vi "Drive type properties.vi"(1 "Type":T1) -> (3 "Nominal resolution":i32, 4 "Effective resolution":dbl, 5 "Rotary":bool, 6 "Speed multiplier":dbl)   [LabVIEW 2019]
uses:
  Axis enum.ctl
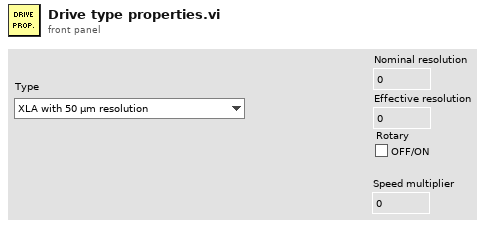
[diagram p1: front panel]
types:
  T1 = typedef "Axis enum.ctl" = enum16{"XLA with 50 µm resolution", "XLA with 10 µm resolution", "XLA with 1250 nm resolution", "XLA with 312 nm resolution", "XLA with 78 nm resolution", "XLS with 1250 nm resolution", "XLS with 312 nm resolution", "XLS with 78nm resolution", "XLS with 5nm resolution", "XLS with 1 nm resolution", "XRT-A with 109 µrad resolution", "XRT-U-30 with 109 µrad resolution", "XRT-U-30 with 49 µrad resolution", "XRT-U-30 with 19 µrad resolution", "XRT-U-30 with 3 µrad resolution", "XRT-U-40 with 109 µrad resolution", "XRT-U 40 with 49 µrad resolution", "XRT-U-40 with 19 µrad resolution", "XRT-U-40 with 3 µrad resolution", "XRT-U-60 with 109 µrad resolution", "XRT-U-60 with 49 µrad resolution", "XRT-U-60 with 19 µrad resolution", "XRT-U-60 with 3 µrad resolution"}
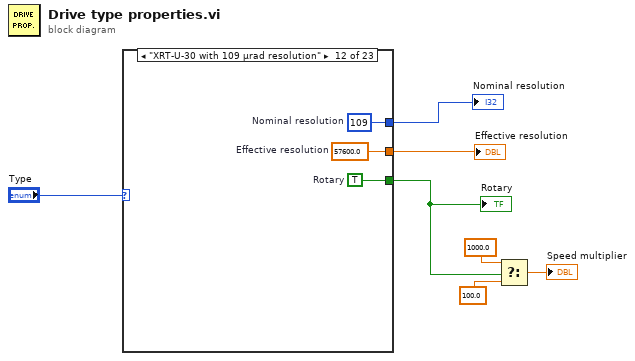
[diagram p0: block diagram]
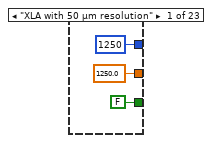
[diagram p2: hidden frame]
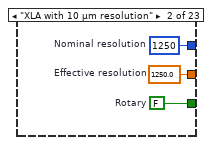
[diagram p3: hidden frame]
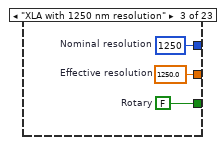
[diagram p4: hidden frame]
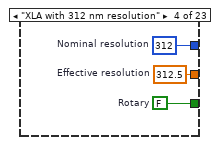
[diagram p5: hidden frame]
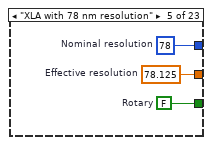
[diagram p6: hidden frame]
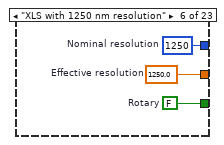
[diagram p7: hidden frame]
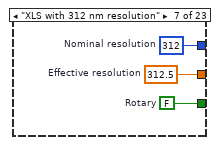
[diagram p8: hidden frame]
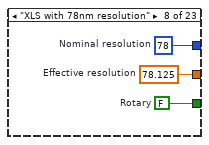
[diagram p9: hidden frame]
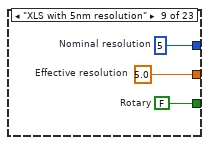
[diagram p10: hidden frame]
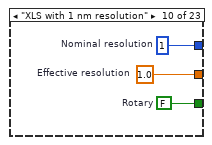
[diagram p11: hidden frame]
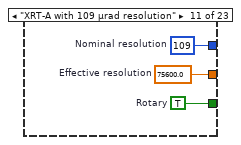
[diagram p12: hidden frame]
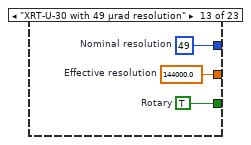
[diagram p13: hidden frame]
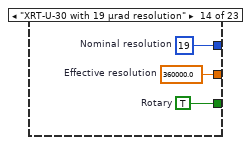
[diagram p14: hidden frame]
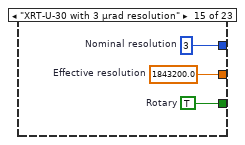
[diagram p15: hidden frame]
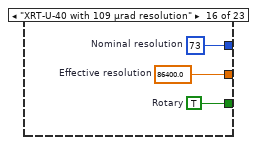
[diagram p16: hidden frame]
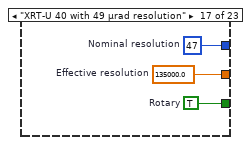
[diagram p17: hidden frame]
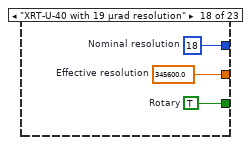
[diagram p18: hidden frame]
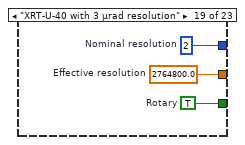
[diagram p19: hidden frame]
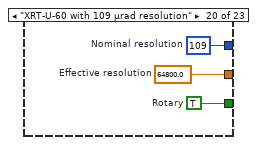
[diagram p20: hidden frame]
diagram:
  n1 = case shown="\"XRT-U-30 with 109 µrad resolution\"" "Type" {
    tunnel: [1250 ("Nominal resolution") w13 w16 w19 w22 w25 w28 w31 w34 w37 w40 w43 w46 w49 w52 w55 w58 w61 w64 w67 w70 w73 w76] -> w6
    tunnel: [1250.0 ("Effective resolution") w12 w15 w18 w21 w24 w27 w30 w33 w36 w39 w42 w45 w48 w51 w54 w57 w60 w63 w66 w69 w72 w75] -> w5
    tunnel: [FALSE ("Rotary") w11 w14 w17 w20 w23 w26 w29 w32 w35 w38 w41 w44 w47 w50 w53 w56 w59 w62 w65 w68 w71 w74] -> w4
    frame "XLA with 50 µm resolution" {
    }
    frame "XLA with 10 µm resolution" {
      w11 = FALSE  # Rotary
      w12 = 1250.0  # Effective resolution
      w13 = 1250  # Nominal resolution
    }
    frame "XLA with 1250 nm resolution" {
      w14 = FALSE  # Rotary
      w15 = 1250.0  # Effective resolution
      w16 = 1250  # Nominal resolution
    }
    frame "XLA with 312 nm resolution" {
      w17 = FALSE  # Rotary
      w18 = 312.5  # Effective resolution
      w19 = 312  # Nominal resolution
    }
    frame "XLA with 78 nm resolution" {
      w20 = FALSE  # Rotary
      w21 = 78.125  # Effective resolution
      w22 = 78  # Nominal resolution
    }
    frame "XLS with 1250 nm resolution" {
      w23 = FALSE  # Rotary
      w24 = 1250.0  # Effective resolution
      w25 = 1250  # Nominal resolution
    }
    frame "XLS with 312 nm resolution" {
      w26 = FALSE  # Rotary
      w27 = 312.5  # Effective resolution
      w28 = 312  # Nominal resolution
    }
    frame "XLS with 78nm resolution" {
      w29 = FALSE  # Rotary
      w30 = 78.125  # Effective resolution
      w31 = 78  # Nominal resolution
    }
    frame "XLS with 5nm resolution" {
      w32 = FALSE  # Rotary
      w33 = 5.0  # Effective resolution
      w34 = 5  # Nominal resolution
    }
    frame "XLS with 1 nm resolution" {
      w35 = FALSE  # Rotary
      w36 = 1.0  # Effective resolution
      w37 = 1  # Nominal resolution
    }
    frame "XRT-A with 109 µrad resolution" {
      w38 = TRUE  # Rotary
      w39 = 75600.0  # Effective resolution
      w40 = 109  # Nominal resolution
    }
    frame "XRT-U-30 with 109 µrad resolution" {
      w41 = TRUE  # Rotary
      w42 = 57600.0  # Effective resolution
      w43 = 109  # Nominal resolution
    }
    frame "XRT-U-30 with 49 µrad resolution" {
      w44 = TRUE  # Rotary
      w45 = 144000.0  # Effective resolution
      w46 = 49  # Nominal resolution
    }
    frame "XRT-U-30 with 19 µrad resolution" {
      w47 = TRUE  # Rotary
      w48 = 360000.0  # Effective resolution
      w49 = 19  # Nominal resolution
    }
    frame "XRT-U-30 with 3 µrad resolution" {
      w50 = TRUE  # Rotary
      w51 = 1843200.0  # Effective resolution
      w52 = 3  # Nominal resolution
    }
    frame "XRT-U-40 with 109 µrad resolution" {
      w53 = TRUE  # Rotary
      w54 = 86400.0  # Effective resolution
      w55 = 73  # Nominal resolution
    }
    frame "XRT-U 40 with 49 µrad resolution" {
      w56 = TRUE  # Rotary
      w57 = 135000.0  # Effective resolution
      w58 = 47  # Nominal resolution
    }
    frame "XRT-U-40 with 19 µrad resolution" {
      w59 = TRUE  # Rotary
      w60 = 345600.0  # Effective resolution
      w61 = 18  # Nominal resolution
    }
    frame "XRT-U-40 with 3 µrad resolution" {
      w62 = TRUE  # Rotary
      w63 = 2764800.0  # Effective resolution
      w64 = 2  # Nominal resolution
    }
    frame "XRT-U-60 with 109 µrad resolution" {
      w65 = TRUE  # Rotary
      w66 = 64800.0  # Effective resolution
      w67 = 109  # Nominal resolution
    }
    frame "XRT-U-60 with 49 µrad resolution" {
      w68 = TRUE  # Rotary
      w69 = 129600.0  # Effective resolution
      w70 = 49  # Nominal resolution
    }
    frame "XRT-U-60 with 19 µrad resolution" {
      w71 = TRUE  # Rotary
      w72 = 324000.0  # Effective resolution
      w73 = 19  # Nominal resolution
    }
    frame "XRT-U-60 with 3 µrad resolution" {
      w74 = TRUE  # Rotary
      w75 = 2073600.0  # Effective resolution
      w76 = 3  # Nominal resolution
    }
  }
  "Nominal resolution" <- w6
  "Effective resolution" <- w5
  "Rotary" <- w4
  n2 = Select(t=1000.0, s=w4, f=100.0) -> (s? t:f=→"Speed multiplier":dbl)
